vi "test Correct Labels In Log.vi"(8 "error in":errorcluster, 11 "TestCase in":refnum<class "Logging Loopback.lvclass">) -> (0 "error out":errorcluster, 3 "TestCase out":refnum<class "Logging Loopback.lvclass">)   [LabVIEW 2020, in "Logging Loopback.lvclass"]
uses:
  Logging Loopback.lvclass
  Logging Loopback.lvclass/Logging Loopback.ctl
  6070ecc1-7a7f-4aba-84f3-8f274e3c644e.vi
  e19d9c75-8616-4056-a7e1-33fbf9884e17.vi
  <vilib>/WebDAVClient/Advanced/Get Buffer.vi
  <vilib>/addons/_JKI Toolkits/VI Tester/TestCase.llb/TestCase.lvclass
  <vilib>/WebDAVClient/NI_WebDAV.lvlib
  C:/Program Files (x86)/National Instruments/LabVIEW 2020/vi.lib/addons/_JKI Toolkits/VI Tester/TestCase.llb/TestCase.lvclass
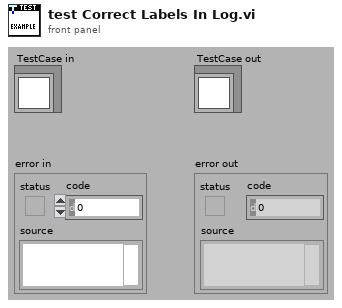
[diagram p1: front panel]
types:
  T1 = typedef "NI_WebDAV.lvlib/SessionHandle.ctl" = refnum<k1>
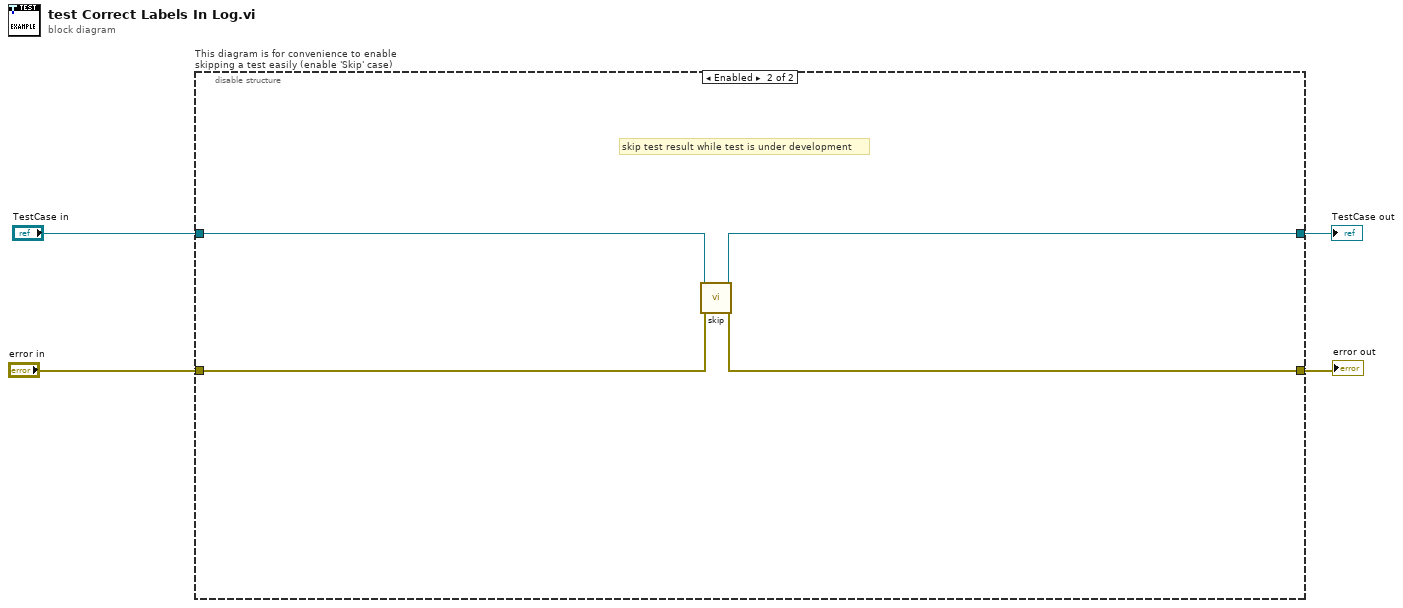
[diagram p0: block diagram]
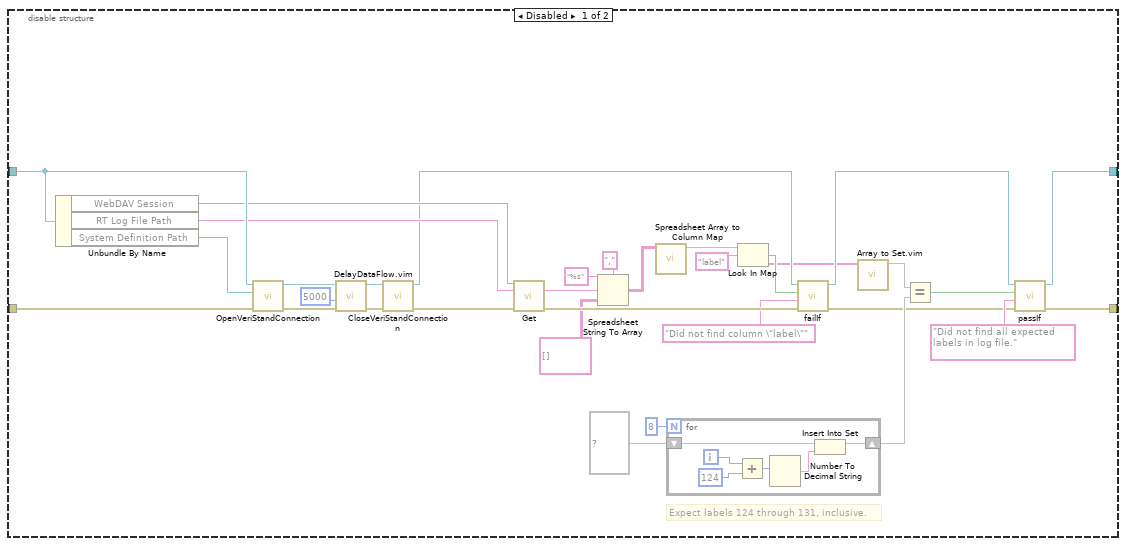
[diagram p2: hidden frame]
diagram:
  n1 = disable-structure "This diagram is for convenience to enable skipping a test easily (enable 'Skip' case)" shown="Enabled" {
    disable-tunnel: "TestCase in" -> [w33 w46]
    disable-tunnel: [w15 w44] -> w1
    disable-tunnel: [w16 w45] -> w3
    disable-tunnel: "error in" -> [w36 w43]
    frame Disabled {
      # "Expect labels 124 through 131, inclusive."
      n2 = Unbundle By Name(w33) -> ("WebDAV Session"=w27:T1, "RT Log File Path"=w26:string, "System Definition Path"=w34:path)
      n3 = call-dynamic "OpenVeriStandConnection.vi"("error in (no error)"=w36, "System Definition File"=w34, "VeriStand Test Case in"=w33) -> ("error out"=w35:errorcluster, "VeriStand Test Case out"=w30:refnum<class "Logging Loopback.lvclass">)  [unwired: 6 in, 1 out]
      n4 = call "DelayDataFlow.vim"("value in"=w35, "milliseconds to wait"=u32 5000) -> ("value out"=w32:errorcluster)  [unwired: 2 in, 1 out]
      n5 = call-dynamic "CloseVeriStandConnection.vi"("error in (no error)"=w32, "VeriStand Test Case in"=w30) -> ("error out"=w29:errorcluster, "VeriStand Test Case out"=w9:refnum<class "Logging Loopback.lvclass">)  [unwired: 8 in]
      n6 = call-poly <vilib>:"Get.vi"("session handle"=w27, "relative uri"=w26, "error in (no error)"=w29) -> ("data"=w25:string, "error out"=w28:errorcluster)  [unwired: 10 in, 1 out]
      n7 = Spreadsheet String To Array(delimiter (Tab)=",", format string="%s", spreadsheet string=w25, array type (2D Dbl)=string[][] []) -> (array=w21:string[][])
      n8 = call "Spreadsheet Array to Column Map.vi"("array"=w21) -> ("map"=w20:map{string, string[]})  [unwired: 10 in]
      n9 = for {
        N: 8 -> [_]
        shift-right: [w41] -> w13
        shift-left: set{string} {} ("set in") -> [w42]
        i -> [w39]
        n10 = Add(x=w39, y=124) -> (x+y=w38:i32)
        n11 = Number To Decimal String(number=w38) -> (decimal integer string=w40:string)  [unwired: 1 in]
        n12 = Insert Into Set(10:w40, 11:w42) -> (3:w41:set{string})  [unwired: 1 out]
      }
      n13 = Look In Map(map=w20, key="label") -> (key not found?=w7:bool, value=w5:string[])  [unwired: 1 in]
      n14 = call-dynamic "failIf.vi"("error in (no error)"=w28, "message (\"\")"="Did not find column \"label\"" ("message (\"\")"), "fail"=w7, "TestCase in"=w9) -> ("error out"=w10:errorcluster, "TestCase out"=w8:refnum<class "Logging Loopback.lvclass">)  [unwired: 6 in]
      n15 = call "Array to Set.vim"("array"=w5) -> ("set"=w14:set{string})  [unwired: 10 in]
      n16 = Equal?(x=w14, y=w13) -> (x = y?=w12:bool)
      n17 = call-dynamic "passIf.vi"("error in (no error)"=w10, "message (\"\")"="Did not find all expected labels in log file." ("message (\"\")"), "pass"=w12, "TestCase in"=w8) -> ("error out"=w16:errorcluster, "TestCase out"=w15:refnum<class "Logging Loopback.lvclass">)  [unwired: 6 in]
    }
    frame Enabled {
      # "skip test result while test is under development"
      n18 = call <vilib>:"skip.vi"("error in (no error)"=w43, "TestCase in"=w46) -> ("error out"=w45:errorcluster, "TestCase out"=w44:refnum<class "Logging Loopback.lvclass">)  [unwired: 8 in]
    }
  }
  "error out" <- w3
  "TestCase out" <- w1
